vi "RF Rec Configure Rx.vi"(0 "niUsrpRio Session":T3={"FPGA Interface"=refnum, "RIO Interface Number"=0, "Data Clock Rate"=0, "FPGA Data Clock Rate"=0, "Global Settings Register Bus"=refnum, "Radio 0 Settings Register Bus"=refnum, "Radio 1 Settings Register Bus"=refnum, "Radio Settings Bus Semaphore"=refnum, "DB Queues"=[], "Characterization Data Valid?"=FALSE, "EEPROM Header"={"Checksum"=0, "Product Code"=0, "Hardware Current Version"=0, "Hardware Oldest Compatible Version"=0, "EEPROM Map Current Version"=0, "EEPROM Map Oldest Compatible Version"=0, "User Password"="", "Pointer to Factory Header"=0, "Pointer to User Header"=0, "Recommended Interval"=0, "Number of Reserved Bytes"=9, "Number of Daughterboards"=0, "Daughterboard IDs"=[], "Daughterboard Serial Numbers"=[]}, "Device Data Header"={"Checksum"=0, "Number of Channels"=0, "Number of Gain Settings"=[], "Pointer to Characterization Data"=[], "Number of Reserved Bytes"=27, "Number of Frequencies"=[]}, "EEPROM Characterization Header"={"Checksum"=0, "Date"=timestamp(0 s since 1904-01-01), "Temperature"=0.0, "Misc. Info"="", "Pointer to Device Data Header"=0, "Number of Reserved Bytes"=28}, "Characterization Data"=[], "FPGA Current Version"=0, "FPGA Oldest Compatible Version"=0, "Fixed Logic Current Version"=0, "Fixed Logic Oldest Compatible Version"=0, "FPGA Radio Settings Bus Current Version"=0, "FPGA Radio Settings Bus Oldest Compatible Version"=0, "FPGA Board Config Current Version"=0, "FPGA Board Config Oldest Compatible Version"=0, "Daughterboard Clock Rate"=0, "daughterboard configuration session handles"=[]} {"Daughterboard Clock Rate" format="%#.3pHz"; "FPGA Data Clock Rate" format="%#.3pHz"; "Data Clock Rate" format="%#.3pHz"; "Characterization Data"."Frequencies [Hz]" format="%#_6p"; "EEPROM Characterization Header"."Pointer to Device Data Header" format="%x"; "EEPROM Characterization Header"."Checksum" format="%x"; "Device Data Header"."Pointer to Characterization Data" format="%x"; "Device Data Header"."Checksum" format="%x"; "EEPROM Header"."Pointer to User Header" format="%x"; "EEPROM Header"."Pointer to Factory Header" format="%x"; "EEPROM Header"."Product Code" format="%x"; "EEPROM Header"."Checksum" format="%x"}, 5 "rx config":T2={"channel configuration"=[], "transfer mode"=enum."Finite", "sample rate"=10000000.0, "number of samples"=8192, "start trigger"=enum."Immediate"} {"channel configuration"."channel configuration"."frequency" format="%#.3pHz"; "channel configuration"."channel configuration"."lo frequency" format="%#.3pHz"; "channel configuration"."channel configuration"."level" format="%#_gdBm"; "sample rate" format="%#.3pS/s"}, 7 "rx.data sink":enum16{"SFP Port 0", "SFP Port 1", "Host"}(ring)=enum."Host", 11 "error in":errorcluster) -> (4 "niUsrpRio Session (out)":T3 {"Daughterboard Clock Rate" format="%#.3pHz"; "FPGA Data Clock Rate" format="%#.3pHz"; "Data Clock Rate" format="%#.3pHz"; "Characterization Data"."Frequencies [Hz]" format="%#_6p"; "EEPROM Characterization Header"."Pointer to Device Data Header" format="%x"; "EEPROM Characterization Header"."Checksum" format="%x"; "Device Data Header"."Pointer to Characterization Data" format="%x"; "Device Data Header"."Checksum" format="%x"; "EEPROM Header"."Pointer to User Header" format="%x"; "EEPROM Header"."Pointer to Factory Header" format="%x"; "EEPROM Header"."Product Code" format="%x"; "EEPROM Header"."Checksum" format="%x"}, 6 "rx.enabled channels":string[](array[string]), 8 "vertical range":dbl[](array[numeric]) format="%#.3pVpp", 14 "rx.coerced configurations":T12 {"coerced sample rates" format="%#.3pS/s"; "coerced levels" format="%#.3gdBm"; "coerced lo frequencies" format="%#.3pHz"; "coerced frequencies" format="%#.3pHz"}, 15 "error out":errorcluster)   [LabVIEW 2018]
uses:
  <instrlib>/niUsrpRio/Config/v1/Host/Public/niUsrpRio Session.ctl
  <instrlib>/_niInstr/Register Bus/v0/Host/Public/Register Bus Session.ctl
  <instrlib>/_niInstr/Register Bus/v0/Host/Private/Session Data.ctl
  <instrlib>/niUsrpRio/Config/v1/Host/Private/DB Queue Reference.ctl
  <instrlib>/niUsrpRio/Config/v1/Host/Private/Daughterboard Data.ctl
  <instrlib>/niUsrpRio/Config/v1/Host/Private/ATR state data.ctl
  <instrlib>/niUsrpRio/Config/v1/Host/Private/Antenna Configuration.ctl
  <instrlib>/niUsrpRio/Config/v1/Host/Private/CPLD Power Mode.ctl
  <instrlib>/niUsrpRio/Config/v1/Host/Public/EEPROM Header.ctl
  <instrlib>/niUsrpRio/Config/v1/Host/Public/EEPROM Device Data Header.ctl
  <instrlib>/niUsrpRio/Config/v1/Host/Public/EEPROM Characterization Header.ctl
  <instrlib>/niUsrpRio/Config/v1/Host/Public/Characterization Data.ctl
  <instrlib>/niUsrpRio/Config/v1/Host/Public/IQ Imbalance.ctl
  RF Rec Start Trigger.ctl
  RF Rec Configure Signal (Level).vi
  <instrlib>/niUsrpRio/Config/v1/Host/niUsrpRio Config v1 Host.lvlib
  <instrlib>/_niInstr/Register Bus/v0/Host/niInstr Register Bus v0 Host.lvlib
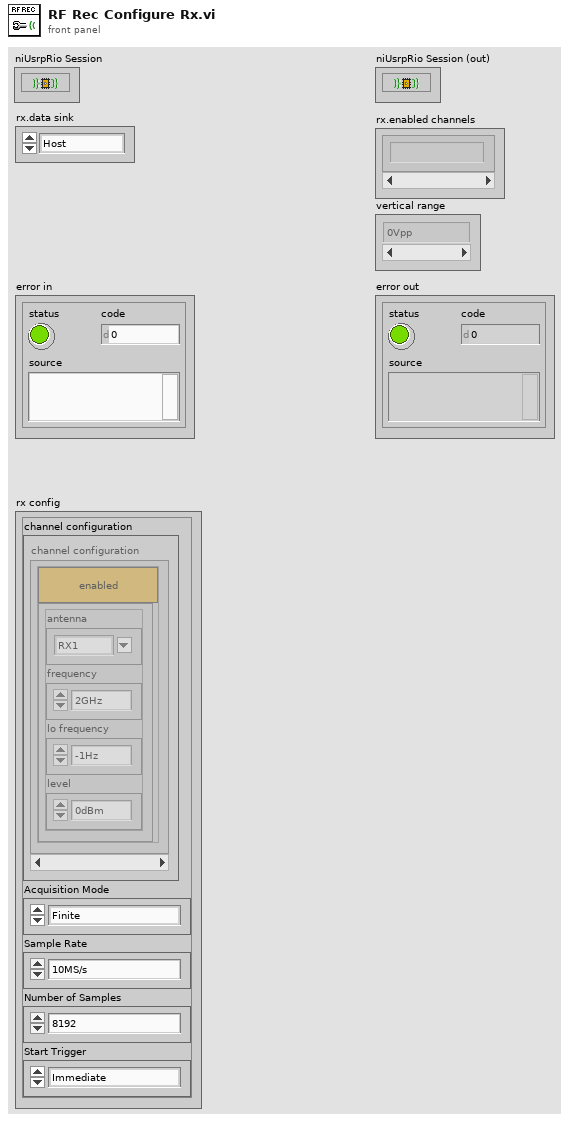
[diagram p1: front panel]
types:
  T1 = typedef "RF Rec Start Trigger.ctl" = enum8{"Software", "Digital Edge", "Rx Start Trigger", "Tx Start Trigger", "Immediate", "Future Time Event"}
  T2 = cluster{"channel configuration":cluster{"channel enable":bool, "channel configuration":cluster{"antenna":string, "frequency":dbl, "lo frequency":dbl, "level":dbl}}[], "transfer mode":enum16{"Finite", "Continuous"}, "sample rate":dbl, "number of samples":u32, "start trigger":T1}
  T3 = typedef "niUsrpRio Config v1 Host.lvlib/niUsrpRio Session.ctl" = cluster{"FPGA Interface":refnum<k20>, "RIO Interface Number":u32, "Data Clock Rate":u32, "FPGA Data Clock Rate":u32, "Global Settings Register Bus":T4, "Radio 0 Settings Register Bus":T4, "Radio 1 Settings Register Bus":T4, "Radio Settings Bus Semaphore":T5, "DB Queues":T6[], "Characterization Data Valid?":bool, "EEPROM Header":T7, "Device Data Header":T8, "EEPROM Characterization Header":T9, "Characterization Data":T10[], "FPGA Current Version":u32, "FPGA Oldest Compatible Version":u32, "Fixed Logic Current Version":u32, "Fixed Logic Oldest Compatible Version":u32, "FPGA Radio Settings Bus Current Version":u32, "FPGA Radio Settings Bus Oldest Compatible Version":u32, "FPGA Board Config Current Version":u32, "FPGA Board Config Oldest Compatible Version":u32, "Daughterboard Clock Rate":u32, "daughterboard configuration session handles":u64[]}
  T4 = typedef "niInstr Register Bus v0 Host.lvlib/Register Bus Session.ctl" = refnum<queue>
  T5 = typedef "Semaphore RefNum" = refnum<k1>
  T6 = typedef "niUsrpRio Config v1 Host.lvlib/DB Queue Reference.ctl" = refnum<queue>
  T7 = typedef "niUsrpRio Config v1 Host.lvlib/EEPROM Header.ctl" = cluster{"Checksum":u32, "Product Code":u16, "Hardware Current Version":u16, "Hardware Oldest Compatible Version":u16, "EEPROM Map Current Version":u16, "EEPROM Map Oldest Compatible Version":u16, "User Password":string, "Pointer to Factory Header":u32, "Pointer to User Header":u32, "Recommended Interval":u16, "Number of Reserved Bytes":i32, "Number of Daughterboards":u8, "Daughterboard IDs":u16[], "Daughterboard Serial Numbers":string[]}
  T8 = typedef "niUsrpRio Config v1 Host.lvlib/EEPROM Device Data Header.ctl" = cluster{"Checksum":u32, "Number of Channels":u8, "Number of Gain Settings":u16[], "Pointer to Characterization Data":u32[], "Number of Reserved Bytes":i32, "Number of Frequencies":u16[]}
  T9 = typedef "niUsrpRio Config v1 Host.lvlib/EEPROM Characterization Header.ctl" = cluster{"Checksum":u32, "Date":timestamp, "Temperature":sgl, "Misc. Info":string, "Pointer to Device Data Header":u32, "Number of Reserved Bytes":i32}
  T10 = typedef "niUsrpRio Config v1 Host.lvlib/Characterization Data.ctl" = cluster{"Gains[dB]":dbl[], "Frequencies [Hz]":dbl[], "IQ Imbalance Table":T11[], "Measured Gains[dB]":dbl[][]}
  T11 = typedef "niUsrpRio Config v1 Host.lvlib/IQ Imbalance.ctl" = cluster{"Gain Imbalance [linear]":dbl, "Phase Imbalance [radians]":dbl, "Offset":cdb}
  T12 = cluster{"coerced frequencies":dbl[], "coerced lo frequencies":dbl[], "coerced levels":dbl[], "coerced sample rates":dbl[]}
  T13 = cluster{"channel enable":bool, "channel configuration":cluster{"antenna":string, "frequency":dbl, "lo frequency":dbl, "level":dbl}}[]
  T14 = cluster{"antenna":string, "frequency":dbl, "lo frequency":dbl, "level":dbl}[]
  T15 = typedef "niUsrpRio Config v1 Host.lvlib/DB Types.ctl" = enum16{"sbx", "cbx", "wbx", "unknown", "ubx", "twinrx"}
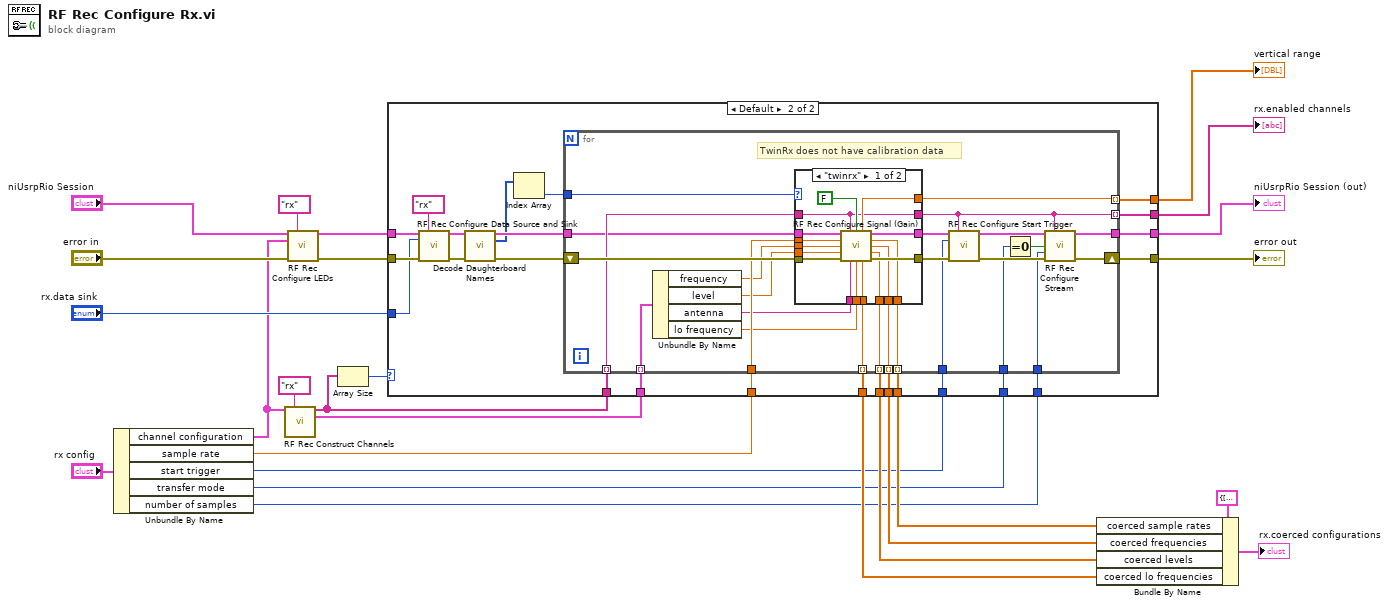
[diagram p0: block diagram]
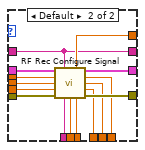
[diagram p3: hidden frame]
diagram:
  n1 = Unbundle By Name("rx config") -> ("channel configuration"=w1:T13, "sample rate"=w10:dbl, "start trigger"=w9:T1, "transfer mode"=w7:enum16{"Finite", "Continuous"}, "number of samples"=w8:u32)
  n2 = call "RF Rec Construct Channels.vi"("channel configurations"=w1, "scope"="rx") -> ("enabled channels"=w13:string[], "enabled channel configurations"=w19:T14)  [unwired: 12 in]
  n3 = call "RF Rec Configure LEDs.vi"("niUsrpRio Session"="niUsrpRio Session", "scope"="rx", "channel configurations"=w1, "error in"="error in") -> ("niUsrpRio Session (out)"=w4:T3, "error out"=w3:errorcluster)  [unwired: 10 in]
  n4 = Array Size(array=w13) -> (size(s)=w14:i32)
  n5 = case shown="Default" w14 {
    tunnel: [_ w52] -> w26
    tunnel: [_ w51] -> w25
    tunnel: [_ w50] -> w24
    tunnel: [_ w49] -> w23
    tunnel: [w28 w48] -> w22
    tunnel: [w27 w47] -> w21
    tunnel: w19 -> [_ w46]
    tunnel: [_ w45] -> w18
    tunnel: [_ w44] -> w15
    tunnel: w10 -> [_ w43]
    tunnel: w9 -> [_ w42]
    tunnel: w7 -> [_ w41]
    tunnel: w8 -> [_ w40]
    tunnel: w3 -> [w27 w38]
    tunnel: w4 -> [w28 w35]
    tunnel: w13 -> [_ w39]
    tunnel: "rx.data sink" -> [_ w37]
    frame 0 {
    }
    frame Default {
      n6 = call "RF Rec Configure Data Source and Sink.vi"("niUsrpRio Session"=w35, "scope"="rx", "data stream config"=w37, "error in"=w38) -> ("niUsrpRio Session (out)"=w34:T3, "error out"=w33:errorcluster)  [unwired: 10 in]
      n7 = call <instrlib>:"Decode Daughterboard Names.vi"("niUsrpRio Session"=w34, "error in"=w33) -> ("niUsrpRio Session (out)"=w32:T3, "daughterboard names"=w30:T15[], "error out"=w31:errorcluster)  [unwired: 10 in, 1 out]
      n8 = Index Array(array=w30) -> (element=w29:T15)  [unwired: 1 in]
      n9 = for "channel configuration" {
        tunnel: [w75] -> w48
        shift-right: [w76] -> w47
        shift-left: w31 -> [w68]
        tunnel: w39 -> [w57] mode=indexing
        tunnel: w46 -> [w74] mode=indexing
        tunnel: [w69] -> w45 mode=indexing
        tunnel: [w73] -> w52 mode=indexing
        tunnel: [w72] -> w51 mode=indexing
        tunnel: [w71] -> w50 mode=indexing
        tunnel: [w70] -> w49 mode=indexing
        tunnel: [w54] -> w44 mode=indexing
        tunnel: w43 -> [w67]
        tunnel: w42 -> [w66]
        tunnel: w41 -> [w65]
        tunnel: w40 -> [w64]
        tunnel: w32 -> [w55]
        tunnel: w29 -> [w53]
        # "TwinRx does not have calibration data"
        n10 = Unbundle By Name(w74) -> ("frequency"=w61:dbl, "level"=w60:dbl, "antenna"=w59:string, "lo frequency"=w58:dbl)
        n11 = case shown="\"twinrx\"" w53 {
          tunnel: [w86 w109] -> w77
          tunnel: [w80 w108] -> w73
          tunnel: [w81 w107] -> w72
          tunnel: [w82 w106] -> w71
          tunnel: [w87 w105] -> w70
          tunnel: [w84 w104] -> w69
          tunnel: w68 -> [w90 w103]
          tunnel: w67 -> [w93 w102]
          tunnel: [w85 w101] -> w62
          tunnel: w61 -> [w92 w100]
          tunnel: w60 -> [w91 w99]
          tunnel: w59 -> [w89 w98]
          tunnel: w58 -> [w88 w97]
          tunnel: w57 -> [w79 w95]
          tunnel: w55 -> [w94 w96]
          tunnel: [w79 w95] -> w54
          frame "twinrx" {
            n12 = call "RF Rec Configure Signal (Gain).vi"("niUsrpRio Session"=w94, "scope"=w79, "Correct Impairments?"=FALSE, "sample rate [S/s]"=w93, "frequency [Hz]"=w92, "gain [dB]"=w91, "error in"=w90, "Active Antenna"=w89, "LO frequency [Hz]"=w88) -> ("cumulative digital gain"=w84:dbl, "niUsrpRio Session (out)"=w85:T3, "coerced sample rate [S/s]"=w80:dbl, "coerced frequency [Hz]"=w81:dbl, "coerced gain [dB]"=w82:dbl, "coerced LO frequency [Hz]"=w87:dbl, "error out"=w86:errorcluster)
          }
          frame Default {
            n13 = call-poly "RF Rec Configure Signal.vi"("niUsrpRio Session"=w96, "scope"=w95, "sample rate [S/s]"=w102, "frequency [Hz]"=w100, "level [dBm]"=w99, "error in"=w103, "Active Antenna"=w98, "LO frequency [Hz]"=w97) -> ("coerced vertical range [Vpp]"=w104:dbl, "niUsrpRio Session (out)"=w101:T3, "coerced sample rate [S/s]"=w108:dbl, "coerced frequency [Hz]"=w107:dbl, "coerced level [dBm]"=w106:dbl, "coerced LO frequency [Hz]"=w105:dbl, "error out"=w109:errorcluster)  [unwired: 1 in]
          }
        }
        n14 = call "RF Rec Configure Start Trigger.vi"("niUsrpRio Session"=w62, "scope"=w54, "start trigger"=w66, "error in"=w77) -> ("niUsrpRio Session (out)"=w63:T3, "error out"=w78:errorcluster)  [unwired: 10 in]
        n15 = Equal To 0?(x=w65) -> (x = 0?=w56:bool)
        n16 = call "RF Rec Configure Stream.vi"("niUsrpRio Session"=w63, "scope"=w54, "number of samples is finite"=w56, "number of samples"=w64, "error in"=w78) -> ("niUsrpRio Session (out)"=w75:T3, "error out"=w76:errorcluster)  [unwired: 9 in]
      }
    }
  }
  "niUsrpRio Session (out)" <- w22
  "error out" <- w21
  "vertical range" <- w18
  "rx.enabled channels" <- w15
  n17 = Bundle By Name(cluster=T12 {"coerced frequencies"=[], "coerced lo frequencies"=[], "coerced levels"=[], "coerced sample rates"=[]} ("coerced configurations"), "coerced sample rates"=w26, "coerced frequencies"=w25, "coerced levels"=w24, "coerced lo frequencies"=w23) -> (→"rx.coerced configurations":T12)
